vi "2HalfAdder.vi"() -> ()   [LabVIEW 2024]
panel:
  in  "z":bool
  out "Carry":bool
  out "Sum":bool
  in  "y":bool
  in  "x":bool
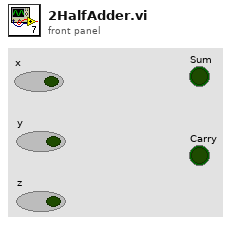
[diagram p1: front panel]
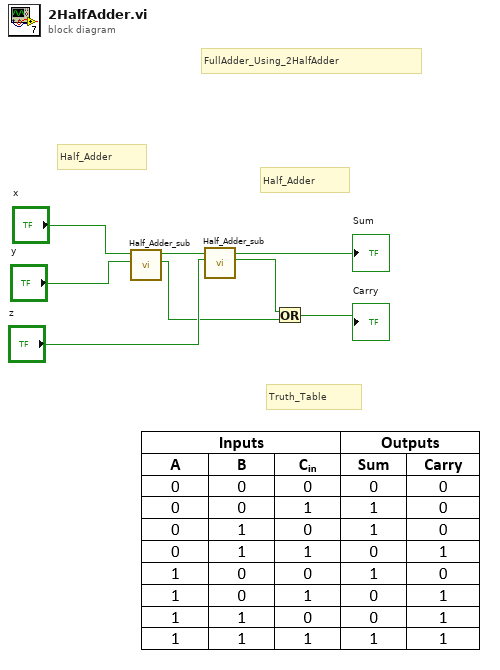
[diagram p0: block diagram]
diagram:
  # "Truth_Table"
  # "FullAdder_Using_2HalfAdder"
  # "Half_Adder"
  # "Half_Adder"
  n1 = call "Half_Adder_sub.vi"("z"="y", "Boolean 3"="x") -> ("Boolean"=w3:bool, "Boolean 2"=w4:bool)  [unwired: 8 in]
  n2 = call "Half_Adder_sub.vi"("z"="z", "Boolean 3"=w4) -> ("Boolean"=w6:bool, "Boolean 2"=→"Sum":bool)  [unwired: 8 in]
  n3 = Or(x=w6, y=w3) -> (x .or. y?=→"Carry":bool)
